vi "Close and Clean Session.vi"(8 "error in":errorcluster, 11 "Session":refnum<class "Session.lvclass">) -> (0 "error out":errorcluster)   [LabVIEW 2015, in "LV-WinSCP.lvlib"]
uses:
  LV-WinSCP.lvlib
  Classes/Session/Session.lvclass
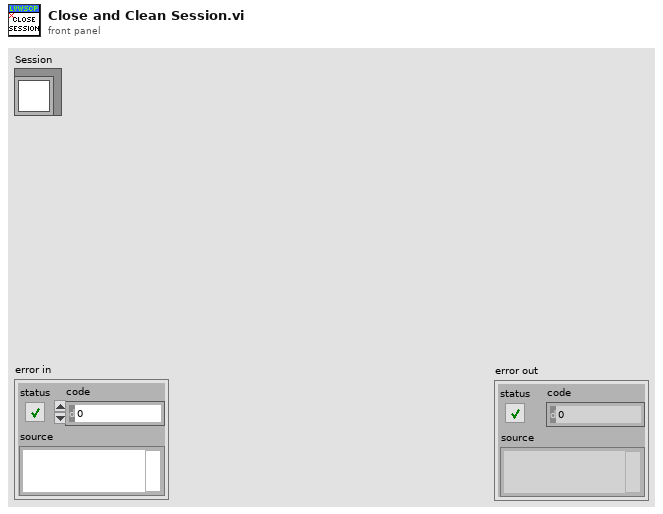
[diagram p1: front panel]
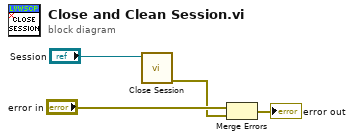
[diagram p0: block diagram]
diagram:
  n1 = call-dynamic "Close Session.vi"("Session in"="Session") -> ("error out"=w1:errorcluster)  [unwired: 10 in]
  n2 = Merge Errors("error in", w1) -> (→"error out":errorcluster)
